vi "Remove Wheel.vi"(8 "error in (no error)":errorcluster, 9 "active wheel indexes in":i32[](array[numeric]), 11 "steering frame ref in":refnum<data-value>) -> (0 "error out":errorcluster, 1 "active wheel indexes out":i32[](array[numeric]), 2 "removed?":bool, 3 "steering frame ref out":refnum<data-value>)   [LabVIEW 2017, in "NI_Robotics_Configure Steering Frame.lvlib"]
uses:
  <vilib>/robotics/Dialog/Configure Steering Frame/NI_Robotics_Configure Steering Frame.lvlib
  <vilib>/robotics/Steering/Steering Frame/NI_Robotics_Steering Frame.lvclass
  <vilib>/robotics/Steering/Steering Frame/NI_Robotics_Steering Frame.lvclass/NI_Robotics_Steering Frame.ctl
  <vilib>/robotics/Utilities/NI_Robotics Utilities.lvlib
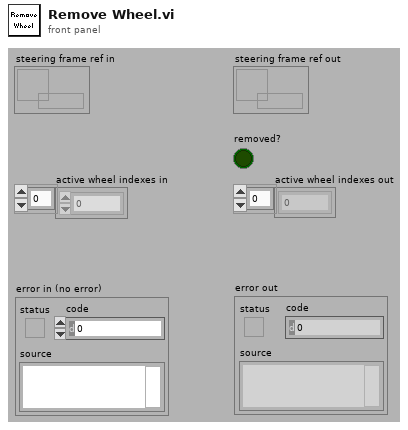
[diagram p1: front panel]
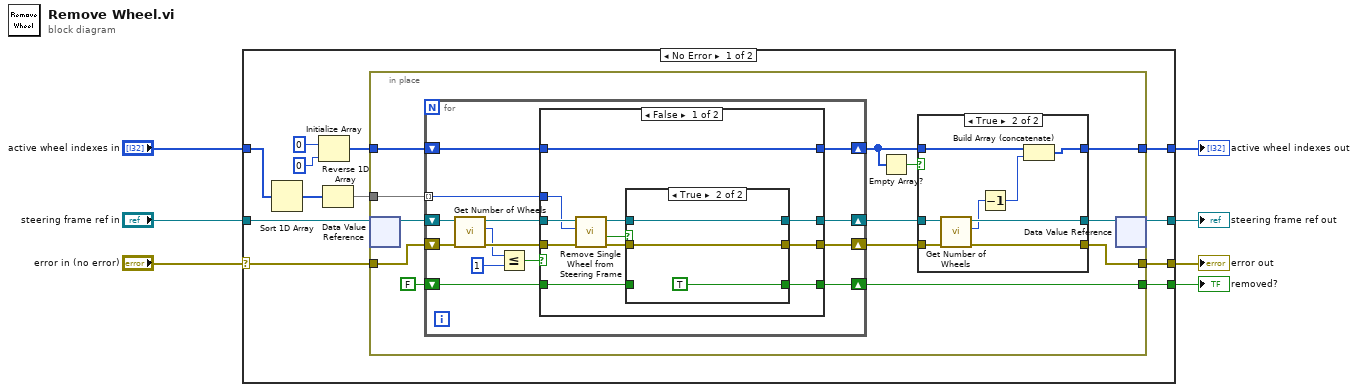
[diagram p0: block diagram]
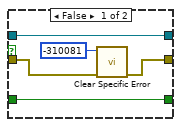
[diagram p3: hidden frame]
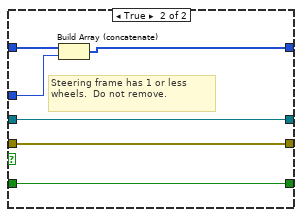
[diagram p4: hidden frame]
diagram:
  n1 = case shown="No Error" "error in (no error)" {
    selector: "error in (no error)" -> [w19 w85]
    tunnel: [w18 w85] -> w6
    tunnel: "steering frame ref in" -> [w17 w83]
    tunnel: "active wheel indexes in" -> [w11 w84]
    tunnel: [w16 w84] -> w4
    tunnel: [w15 w83] -> w3
    tunnel: [w14 _] -> w2
    frame No Error {
      n2 = Sort 1D Array(array=w11) -> (sorted array=w13:i32[])
      n3 = Initialize Array(0 ("Numeric"), 0 ("dimension size")) -> (w8:i32[])
      n4 = Reverse 1D Array(array=w13) -> (reversed array=w12:i32[])
      n5 = in-place {
        in-place-border: w19 -> [w30]
        in-place-border: [w22] -> w18
        in-place-border: [w26] -> w16
        in-place-border: [w20] -> w14
        in-place-border: w12 -> [w31]
        in-place-border: w8 -> [w29]
        n6 = in-place-dvr #1(w17) -> (w32:refnum<class "NI_Robotics_Steering Frame.lvclass">)  [unwired: 1 out]
        n7 = for {
          shift-right: [w48] -> w25
          shift-left: w32 -> [w57]
          tunnel: w31 -> [w51] mode=indexing
          shift-right: [w47] -> w23
          shift-left: w30 -> [w56]
          shift-right: [w49] -> w27
          shift-left: w29 -> [w50]
          shift-right: [w45] -> w20
          shift-left: FALSE -> [w44]
          n8 = call <vilib>:"Get Number of Wheels.vi"("error in (no error)"=w56, "steering frame in"=w57) -> ("error out"=w52:errorcluster, "number of wheels"=w46:i32, "steering frame out"=w53:refnum<class "NI_Robotics_Steering Frame.lvclass">)  [unwired: 7 in]
          n9 = Less Or Equal?(x=w46, y=1) -> (x <= y?=w54:bool)
          n10 = case shown="False" w54 {
            tunnel: w53 -> [w68 w79]
            tunnel: w52 -> [w67 w78]
            tunnel: w51 -> [w66 w81]
            tunnel: w50 -> [w60 w82]
            tunnel: [w60 w80] -> w49
            tunnel: [w63 w79] -> w48
            tunnel: [w61 w78] -> w47
            tunnel: [w59 w77] -> w45
            tunnel: w44 -> [w58 w77]
            frame False {
              n11 = call <vilib>:"Remove Single Wheel from Steering Frame.vi"("error in (no error)"=w67, "wheel index"=w66, "steering frame in"=w68) -> ("error out"=w62:errorcluster, "found?"=w65:bool, "steering frame out"=w64:refnum<class "NI_Robotics_Steering Frame.lvclass">)  [unwired: 2 in, 4 out]
              n12 = case shown="True" w65 {
                tunnel: w64 -> [w73 w76]
                tunnel: w62 -> [w71 w75]
                tunnel: [w73 w76] -> w63
                tunnel: [w70 w75] -> w61
                tunnel: [w69 TRUE] -> w59
                tunnel: w58 -> [w69 _]
                frame False {
                  n13 = call <vilib>:"Clear Specific Error.vi"("error in (no error)"=w71, "code"=-310081) -> ("error out"=w70:errorcluster)  [unwired: 7 in, 2 out]
                }
                frame True {
                }
              }
            }
            frame True {
              # "Steering frame has 1 or less wheels.  Do not remove."
              n14 = Build Array (concatenate)(w82, w81) -> (w80:i32[])
            }
          }
        }
        n15 = Empty Array?(array=w27) -> (empty?=w28:bool)
        n16 = case shown="True" w28 {
          tunnel: w27 -> [w35 w38]
          tunnel: [w35 w36] -> w26
          tunnel: w25 -> [w34 w42]
          tunnel: [w34 w41] -> w24
          tunnel: w23 -> [w33 w43]
          tunnel: [w33 w40] -> w22
          frame False {
          }
          frame True {
            n17 = call <vilib>:"Get Number of Wheels.vi"("error in (no error)"=w43, "steering frame in"=w42) -> ("error out"=w40:errorcluster, "number of wheels"=w39:i32, "steering frame out"=w41:refnum<class "NI_Robotics_Steering Frame.lvclass">)  [unwired: 7 in]
            n18 = Decrement(x=w39) -> (x-1=w37:i32)
            n19 = Build Array (concatenate)(w38, w37) -> (w36:i32[])
          }
        }
        n20 = in-place-dvr #1(w24) -> (w15:refnum<data-value>)  [unwired: 1 out]
      }
    }
    frame Error {
    }
  }
  "error out" <- w6
  "steering frame ref out" <- w3
  "active wheel indexes out" <- w4
  "removed?" <- w2
